vi "NLRBeobachter.vi"(0 "x1":dbl, 1 "x3":dbl, 2 "u":dbl) -> (20 "x1_":dbl, 21 "x2_":dbl, 22 "x3_":dbl, 23 "x4_":dbl[](array[numeric]), 24 "Differenz_x1":dbl)   [LabVIEW 2013]
uses:
  <vilib>/Simulation/Scripting/Companion Diagram/SimConfigNode/SimDog.xnode
  <vilib>/Simulation/Implementation/Shared/SIMSCR Execution Mode.ctl
  <vilib>/Simulation/Scripting/Companion Diagram/SimConfigNode/_simSolvers.ctl
  <vilib>/Simulation/Scripting/Companion Diagram/SimConfigNode/SimParams.ctl
  x4_.vi
  f24.vi
  f23.vi
  f44.vi
  f43.vi
  x3_.vi
  F.vi
  diff_x1.vi
  L21.vi
  L11.vi
  L41.vi
  L42.vi
  diff_x3.vi
  L31.vi
  L32.vi
  <vilib>/Simulation/Implementation/XNodeFramework/SimXNode/SimX.xnode
  <vilib>/Simulation/SignalArithmetic/Implementation/NILVSim Gain.llb/SIM Gain (scalar).vi
  <vilib>/Simulation/ContinuousLinear/Implementation/NILVSim Integrator new.llb/SIM Integrator (scalar).vi
  <vilib>/Simulation/SignalDisplay/Implementation/NILVSim Time Waveform.llb/SIM Time Waveform (scalar).vi
  Root.vi
  Root1.vi
  d(f2+g2u)_dx3.vi
  d(f2+g2u)_dx4.vi
  d(f4+g4u)_dx3.vi
  d(f4+g4u)_dx4.vi
  f2+g2u.vi
  f4+g4u.vi
  <vilib>/Simulation/SignalDisplay/Implementation/NILVSim Time Waveform.llb/SIM Time Waveform (vector).vi
  <vilib>/Simulation/ContinuousLinear/Implementation/NILVSim Integrator new.llb/SIM Integrator (vector).vi
  <vilib>/Simulation/Nonlinear/Implementation/NILVSim Saturation.llb/SIM Saturation (scalar).vi
panel:
  out "Scope9":waveform(dbl)[](graph)
  out "Scope8":waveform(dbl)(graph)
  out "Scope7":waveform(dbl)(graph)
  out "Scope6":waveform(dbl)[](graph)
  out "Scope5":waveform(dbl)(graph)
  out "Scope4":waveform(dbl)[](graph)
  out "Scope3":waveform(dbl)[](graph)
  out "Scope2":waveform(dbl)(graph)
  out "Scope1":waveform(dbl)(graph)
  out "Scope":waveform(dbl)[](graph)
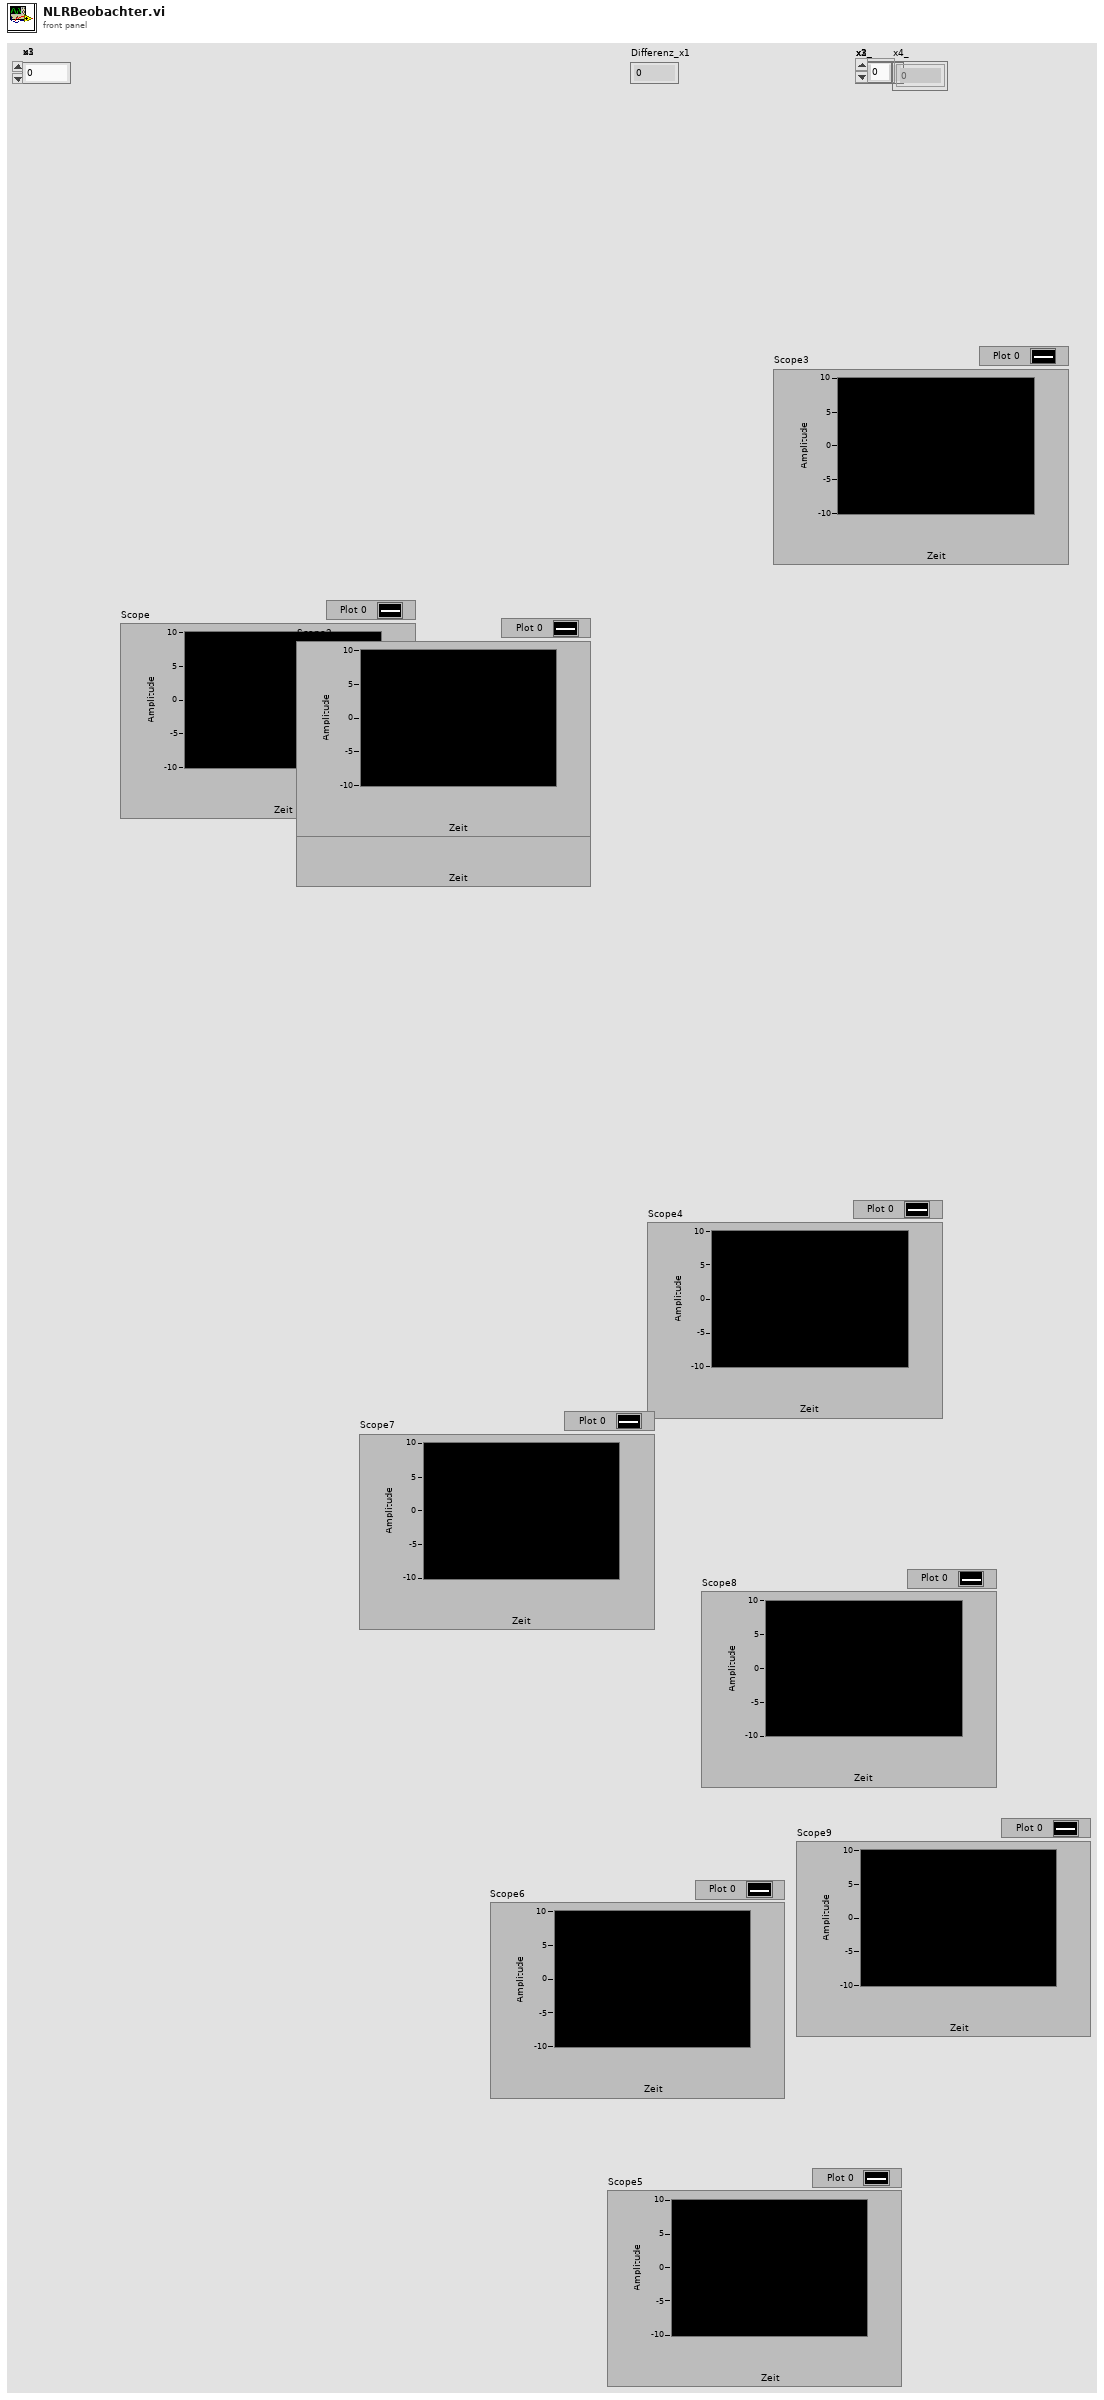
[diagram p1: front panel]
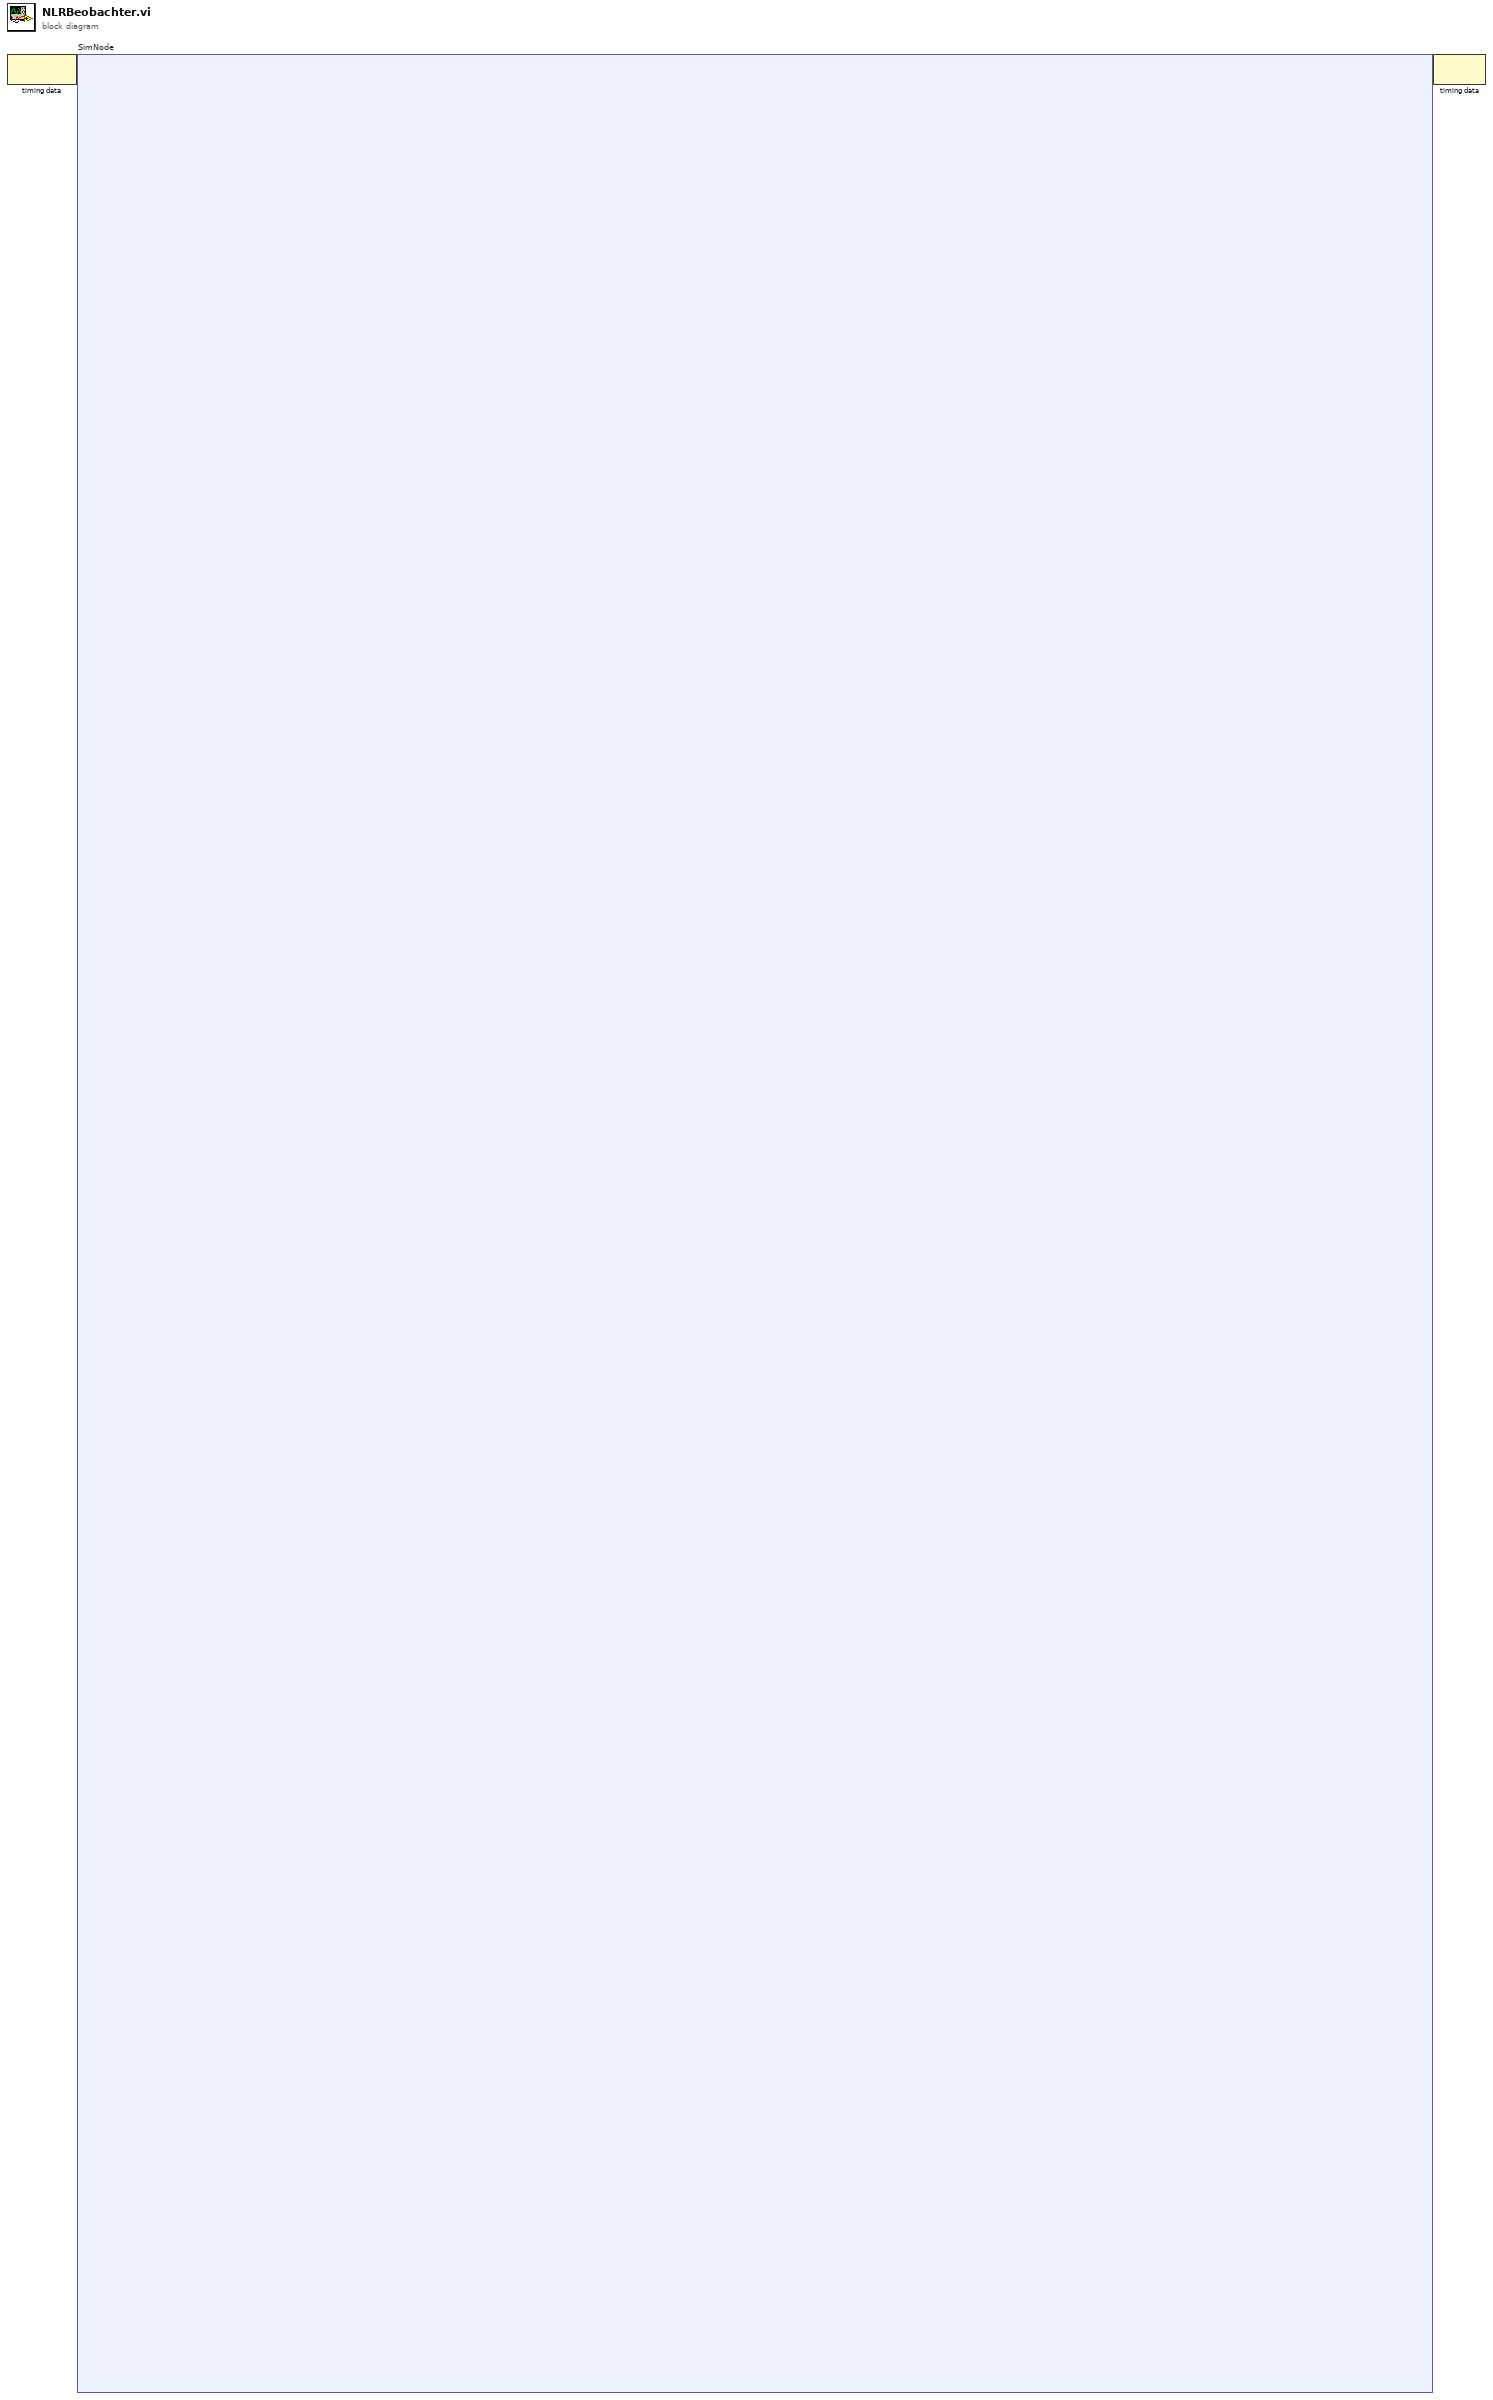
[diagram p0: block diagram]
diagram:
  n1 = node-c288() -> (w2:variant)  [unwired: 1 in]
  n2 = node-c254 "SimNode"(w2) -> (w1:variant)
  n3 = node-c288(w1) -> ()  [unwired: 1 out]
